vi "onStop.vi"(8 "error in (no error)":errorcluster, 11 "Client in":refnum<class "Client.lvclass">) -> (0 "error out":errorcluster, 3 "Client out":refnum<class "Client.lvclass">)   [LabVIEW 2013, in "MQTT Client.lvlib" / "Client.lvclass"]
uses:
  Client.lvclass
  Client.lvclass/Client.ctl
  <vilib>/LabVIEW Open Source Project/MQTT Connection/MQTT_Base/Base Class/MQTT_Base.lvclass
  <vilib>/LabVIEW Open Source Project/MQTT Control Packets/Control Packets/PUBLISH/PUBLISH.lvclass
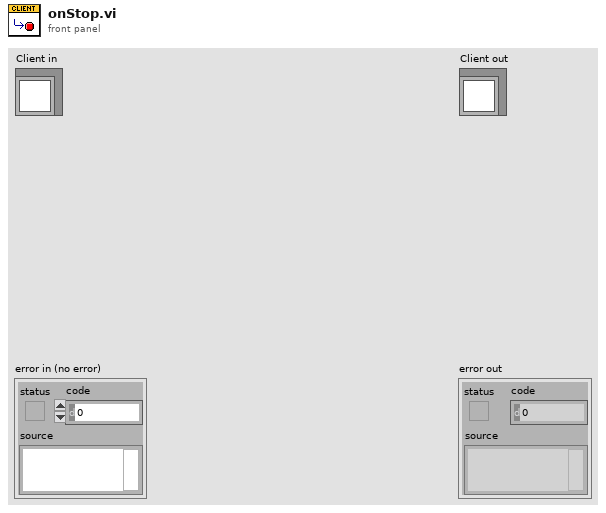
[diagram p1: front panel]
types:
  T1 = typedef "MQTT Client.lvlib/Client.lvclass/Public Events -- cluster.ctl" = cluster{"Connection Status":refnum<user-event>, "Connected":refnum<user-event>, "Application Message":refnum<user-event>}
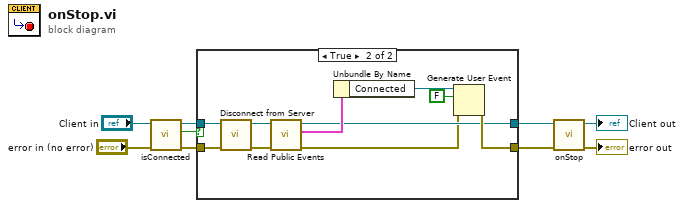
[diagram p0: block diagram]
diagram:
  n1 = call "isConnected.vi"("error in (no error)"="error in (no error)", "Client in"="Client in") -> ("error out"=w4:errorcluster, "connected"=w1:bool, "Client out"=w2:refnum<class "Client.lvclass">)  [unwired: 7 in]
  n2 = case shown="True" w1 {
    tunnel: [w10 w20] -> w7
    tunnel: [w11 w16] -> w6
    tunnel: w4 -> [w10 w13]
    tunnel: w2 -> [w11 w12]
    frame False {
    }
    frame True {
      n3 = call "Disconnect from Server.vi"("error in (no error)"=w13, "Client in"=w12) -> ("error out"=w15:errorcluster, "Client out"=w17:refnum<class "Client.lvclass">)  [unwired: 7 in, 1 out]
      n4 = call "Read Public Events.vi"("error in (no error)"=w15, "Client in"=w17) -> ("error out"=w14:errorcluster, "Client Public Events"=w18:T1, "Client out"=w16:refnum<class "Client.lvclass">)  [unwired: 7 in]
      n5 = Unbundle By Name(w18) -> ("Connected"=w21:refnum<user-event>)
      n6 = Generate User Event(user event=w21, event data cluster=FALSE ("event data"), error in=w14) -> (error out=w20:errorcluster)  [unwired: 1 in, 1 out]
    }
  }
  n7 = call-parent "onStop.vi"("error in (no error)"=w7, "MQTT_Base in"=w6) -> ("error out"=→"error out":errorcluster, "MQTT_Base out"=→"Client out":refnum<class "Client.lvclass">)  [unwired: 8 in]
